vi "SpaceInvaders.vi"() -> ()   [LabVIEW 2022 SP3]
uses:
  TransPicture.ctl
  SelectKb.ctl
  ShipShootEnum.ctl
  InvaderPositionArray.ctl
  move_dir_lr.ctl
  ShotCluster.ctl
  move_dir_ud.ctl
  <vilib>/Utility/error.llb/Trim Whitespace One-Sided.vi
  Globals.vi
panel:
  out "ShootEnergy":dbl(slide) scale=0.0..500.0
  out "Intensity_DP":u8[][](graph)
  out "Ship":T1
  out "Invaders":T1
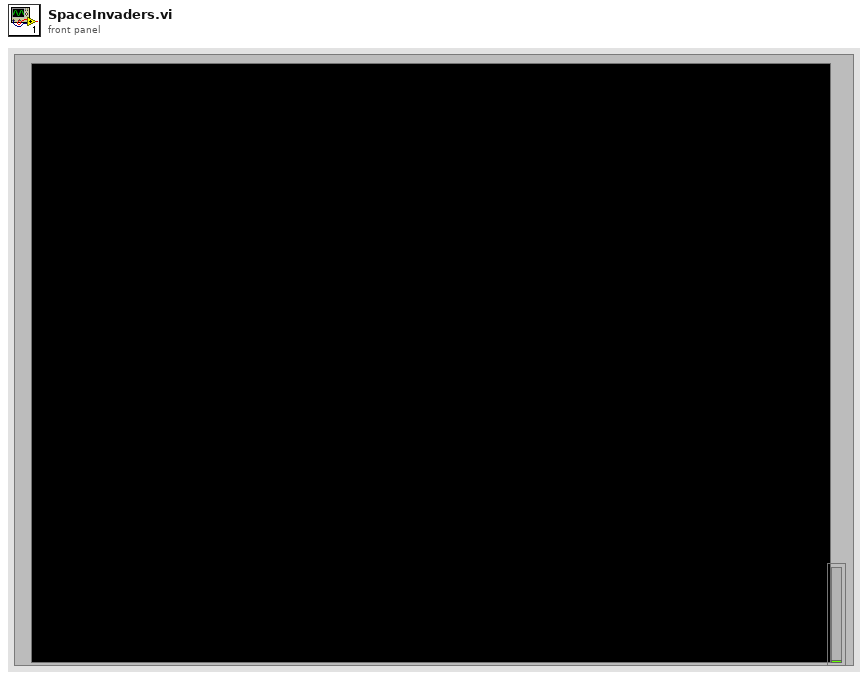
[diagram p1: front panel]
types:
  T1 = typedef "TransPicture.ctl" = picture
  T2 = typedef "ShipShootEnum.ctl" = enum16{"Init", "Read", "Reset"}
  T3 = typedef "SelectKb.ctl" = enum16{"InitKeyboard", "GetPressedKeys"}
  T4 = enum16{"0", "1", "2", "3", "4", "5", "6", "7", "8", "9", "A", "B", "C", "D", "E", "F", "G", "H", "I", "J", "K", "L", "M", "N", "O", "P", "Q", "R", "S", "T", "U", "V", "W", "X", "Y", "Z", "F1", "F2", "F3", "F4", "F5", "F6", "F7", "F8", "F9", "F10", "F11", "F12", "F13", "F14", "F15", "ADD", "BACK", "BACKSLASH", "CAPITAL", "COMMA", "DECIMAL", "DELETE", "DIVIDE", "DOWN", "END", "EQUALS", "ESCAPE", "GRAVE (`)", "HOME", "INSERT", "LBRACKET", "LCONTROL", "LEFT", "L ALT", "LSHIFT", "LWIN", "MINUS", "MULTIPLY", "NEXT", "NUMLOCK", "NUMPAD_0", "NUMPAD_1", "NUMPAD_2", "NUMPAD_3", "NUMPAD_4", "NUMPAD_5", "NUMPAD_6", "NUMPAD_7", "NUMPAD_8", "NUMPAD_9", "PAUSE", "PERIOD", "PRIOR (PG UP)", "RBRACKET", "RCONTROL", "RETURN", "RIGHT", "R ALT", "RSHIFT", "RWIN", "SCROLL", "SEMICOLON", "SLASH", "SPACE", "SUBTRACT", "TAB", "UP", "ENTER (num pad)", "' (quote)"}
  T5 = enum32{"Invalid", "Standard", "Closed", "Hidden", "Minimized", "Maximized"}
  T6 = enum32{"invalid app kind", "Development System", "Run Time System", "Student Edition", "Embedded LabVIEW", "Evaluation", "Custom"}
  T7 = typedef "move_dir_lr.ctl" = enum16{"right", "left"}
  T8 = typedef "InvaderPositionArray.ctl" = cluster{"InvaderAlive":bool[][], "InvaderPosArray":cluster{"left":i16, "top":i16, "right":i16, "bottom":i16}[][], "Direction":T7}
  T9 = typedef "move_dir_ud.ctl" = enum16{"up", "down"}
  T10 = typedef "ShotCluster.ctl" = cluster{"Speed":u32, "Length":u32, "Width":u32, "Position":cluster{"left":i16, "top":i16, "right":i16, "bottom":i16}, "Direction":T9}
  T11 = enum16{"0", "1", "2", "3", "4", "5", "6", "7", "8", "9", "A", "B", "C", "D", "E", "F", "G", "H", "I", "J", "K", "L", "M", "N", "O", "P", "Q", "R", "S", "T", "U", "V", "W", "X", "Y", "Z", "F1", "F2", "F3", "F4", "F5", "F6", "F7", "F8", "F9", "F10", "F11", "F12", "F13", "F14", "F15", "ADD", "BACK", "BACKSLASH", "CAPITAL", "COMMA", "DECIMAL", "DELETE", "DIVIDE", "DOWN", "END", "EQUALS", "ESCAPE", "GRAVE (`)", "HOME", "INSERT", "LBRACKET", "LCONTROL", "LEFT", "L ALT", "LSHIFT", "LWIN", "MINUS", "MULTIPLY", "NEXT", "NUMLOCK", "NUMPAD_0", "NUMPAD_1", "NUMPAD_2", "NUMPAD_3", "NUMPAD_4", "NUMPAD_5", "NUMPAD_6", "NUMPAD_7", "NUMPAD_8", "NUMPAD_9", "PAUSE", "PERIOD", "PRIOR (PG UP)", "RBRACKET", "RCONTROL", "RETURN", "RIGHT", "R ALT", "RSHIFT", "RWIN", "SCROLL", "SEMICOLON", "SLASH", "SPACE", "SUBTRACT", "TAB", "UP", "ENTER (num pad)", "' (quote)"}[]
  T12 = typedef "InitCluster.ctl" = cluster{"Invader":T13, "Spaceship":T13, "game_screen":refnum<vi>, "BasePicture":picture, "invader_screen":refnum<vi>, "InvaderPicPosition":T16, "Invader_down_speed":i16, "FPS":u16, "InvaderBlockSize":T17, "ship_screen":refnum<vi>, "ShipBlockSize":T17, "ShipPicPosition":T16, "LastUpdate":u32, "Intensity_Dp":refnum<vi>, "IntensityArray":u8[][], "ShotArray":T10[], "InvaderShotTimeArray":u32[], "ShootPeriod_ms":i32, "LastShipShot":u32}
  T13 = typedef "CharacterCluster.ctl" = cluster{"image":T14, "Width":u32, "Hieght":u32, "SpeedCharacter":u32, "Shot":T15, "IntensityArray":u8[][]}
  T14 = typedef "imagedata.ctl" = cluster{"image type":i32, "image depth":i32, "image":u8[], "mask":u8[], "colors":u32[], "Rectangle":cluster{"left":i16, "top":i16, "right":i16, "bottom":i16}}
  T15 = typedef "ShotInitCluster.ctl" = cluster{"Speed":u32, "Length":u32, "Width":u32}
  T16 = typedef "LVPositionTypeDef.ctl" = cluster{"Left":i32, "Top":i32}
  T17 = typedef "LVBoundsTypeDef.ctl" = cluster{"Width":u32, "Height":u32}
  T18 = cluster{"Core":cluster{"Current VI Reference":refnum<vi>, "Close Panel on Exit?":bool}, "InitCluster":T12, "InvaderPosArray":T8, "SpaceshipPosition":cluster{"left":i16, "top":i16, "right":i16, "bottom":i16}}
  T19 = cluster{"left":i16, "top":i16, "right":i16, "bottom":i16}
  T20 = cluster{"Current VI Reference":refnum<vi>, "Close Panel on Exit?":bool}
  T21 = cluster{"left":i16, "top":i16, "right":i16, "bottom":i16}[][]
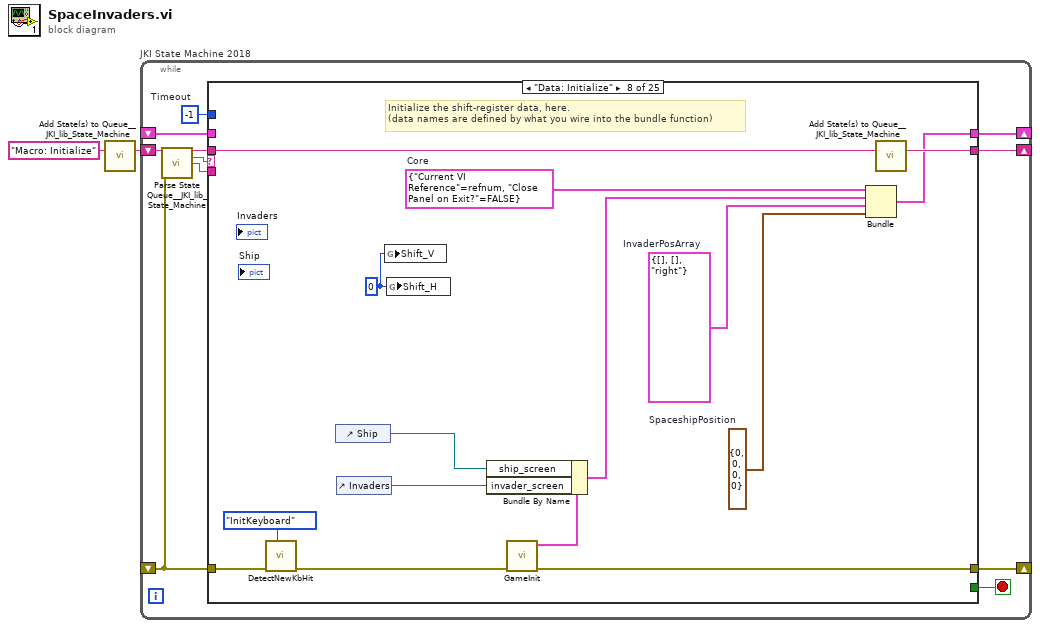
[diagram p0: block diagram]
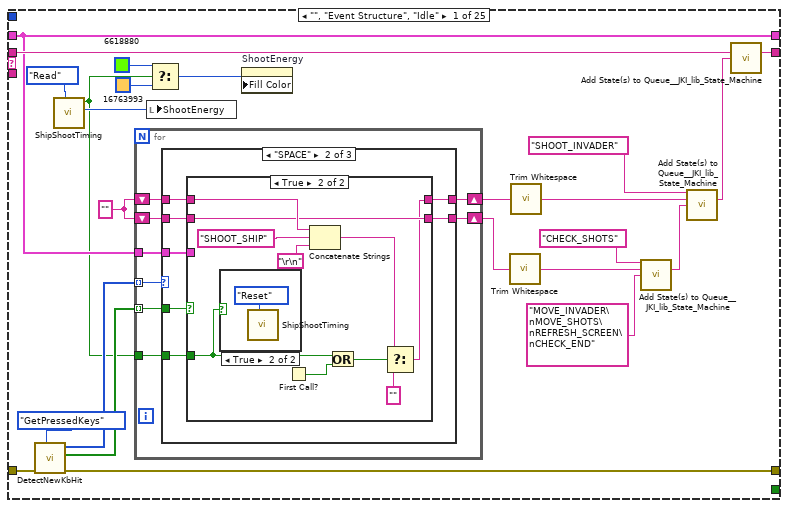
[diagram p2: hidden frame]
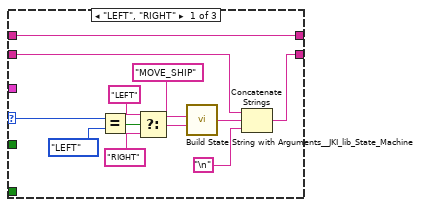
[diagram p3: hidden frame]
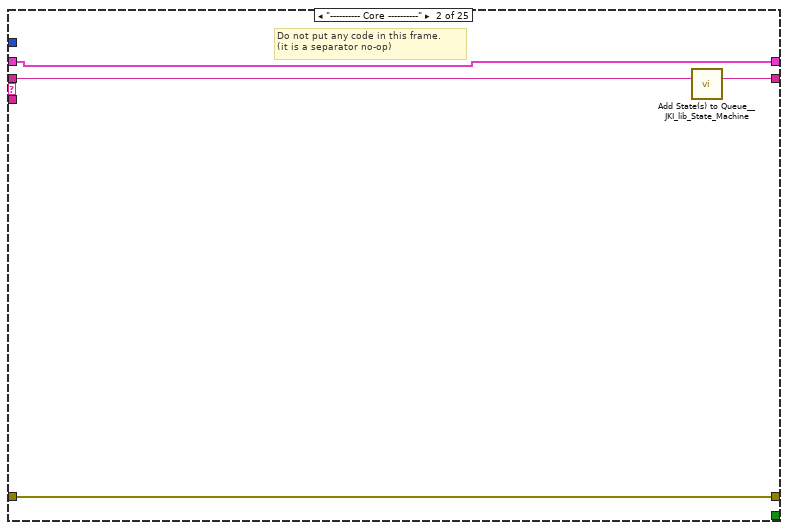
[diagram p7: hidden frame]
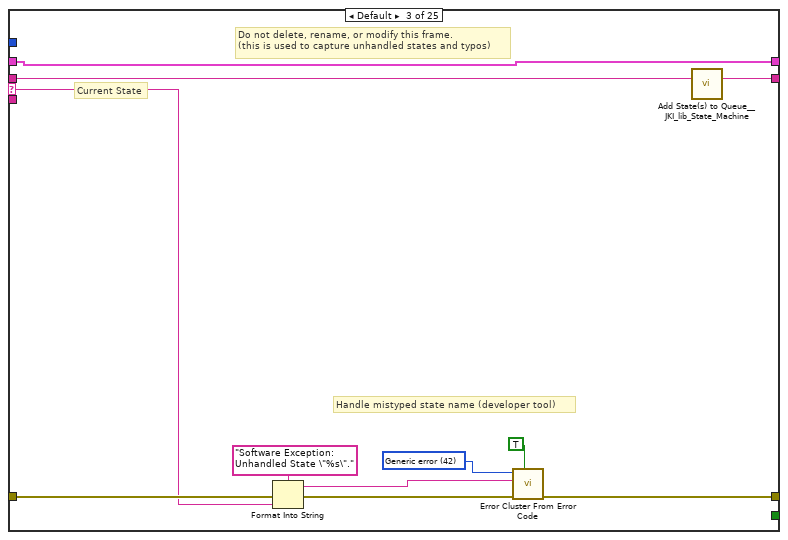
[diagram p8: hidden frame]
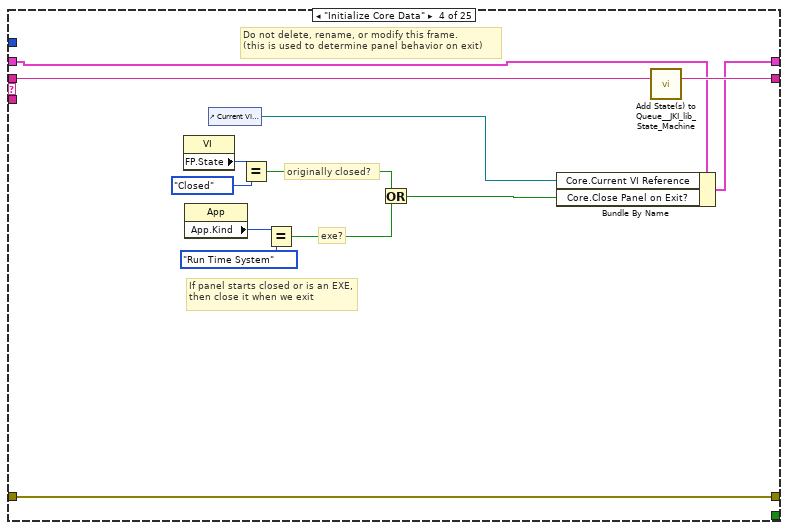
[diagram p9: hidden frame]
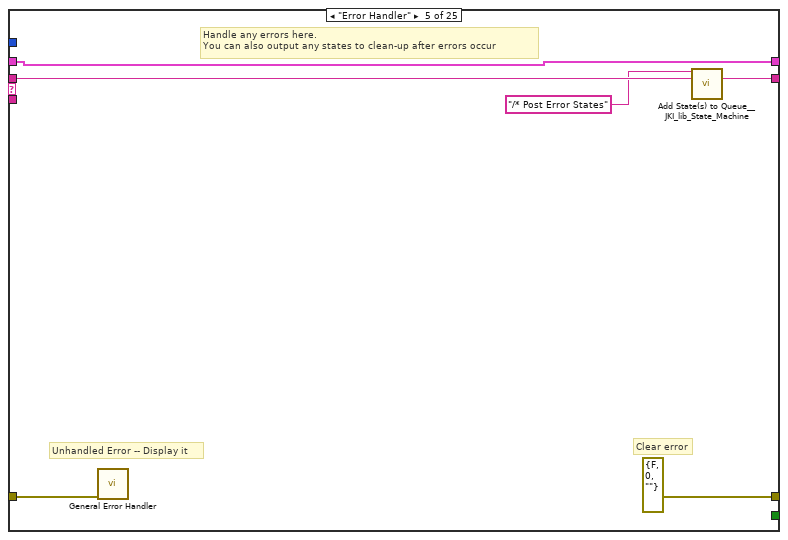
[diagram p10: hidden frame]
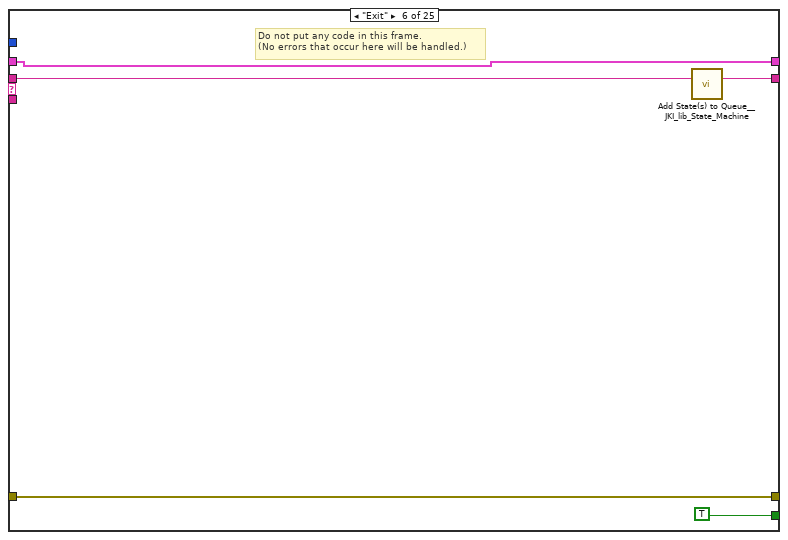
[diagram p11: hidden frame]
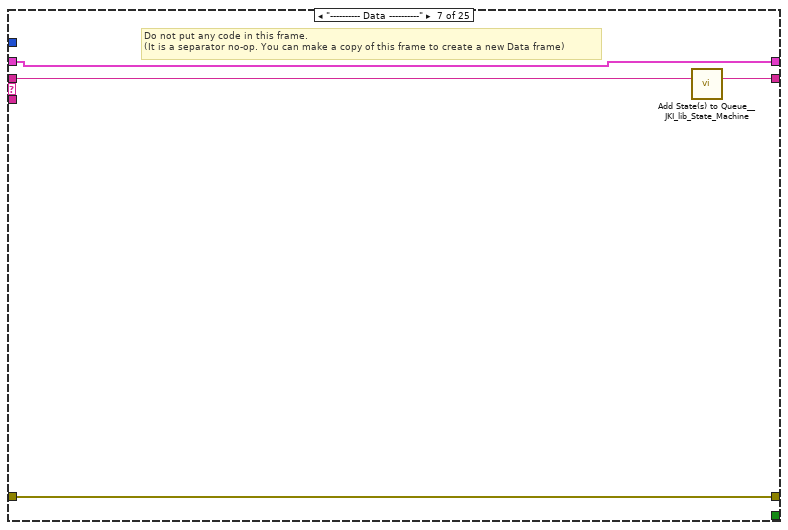
[diagram p12: hidden frame]
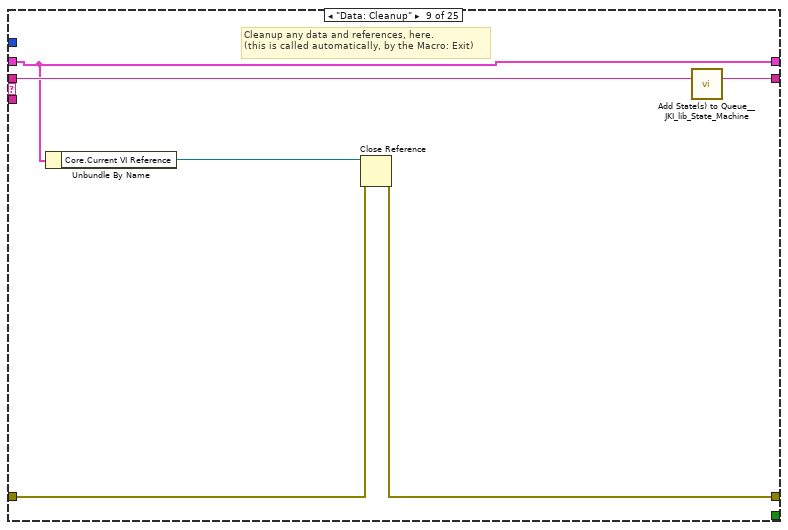
[diagram p13: hidden frame]
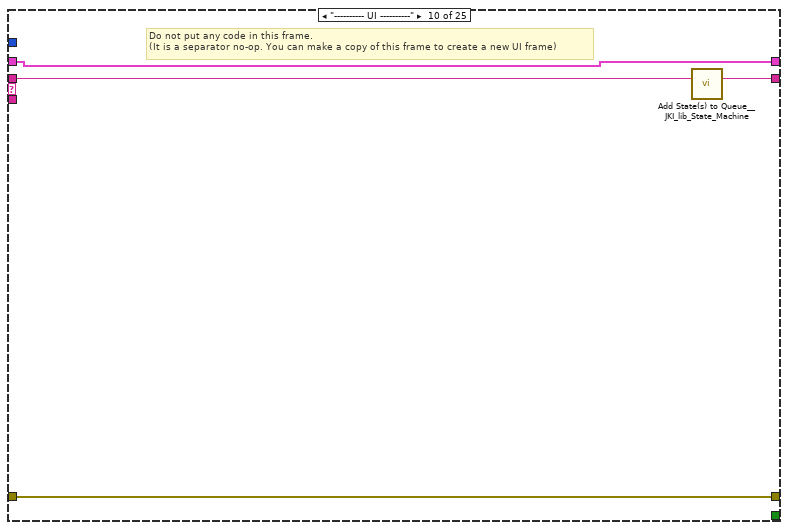
[diagram p14: hidden frame]
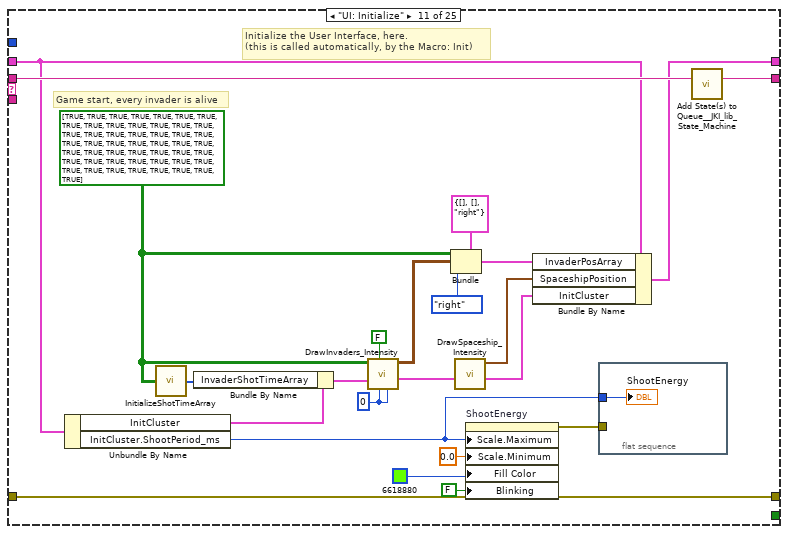
[diagram p15: hidden frame]
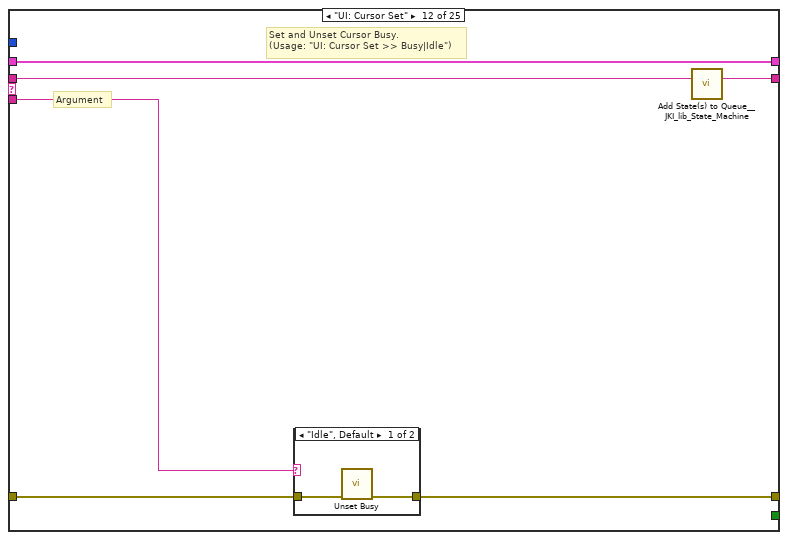
[diagram p16: hidden frame]
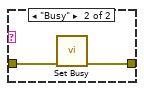
[diagram p17: hidden frame]
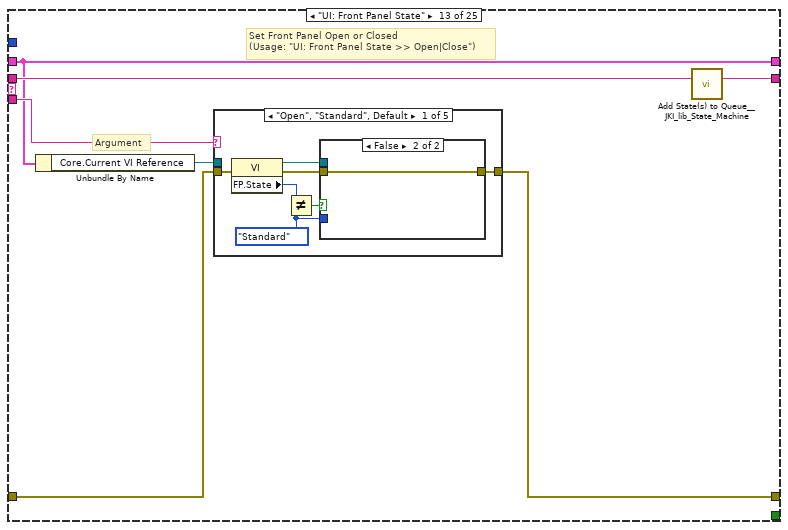
[diagram p18: hidden frame]
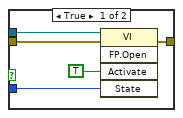
[diagram p19: hidden frame]
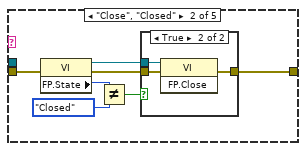
[diagram p20: hidden frame]
diagram:
  n1 = call <vilib>:"Add State(s) to Queue__JKI_lib_State_Machine.vi"("State(s) in (\"\")"="Macro: Initialize") -> ("States Out"=w2:string)  [unwired: 14 in]
  n2 = while "JKI State Machine 2018" {
    shift-right: [w6] -> _
    shift-left: _ -> [w3]
    shift-right: [w9] -> _
    shift-left: _ -> [w4]
    shift-right: [w8] -> _
    shift-left: w2 -> [w10]
    stop <- w7 stop-if-true
    w5 = -1  # Timeout
    n3 = call <vilib>:"Parse State Queue__JKI_lib_State_Machine.vi"("State Queue"=w10, "Error In (no error)"=w4) -> ("Remaining States"=w12:string, "Current State"=w13:string, "Arguments"=w11:string)  [unwired: 11 in]
    n4 = case shown="\"Data: Initialize\"" w13 {
      selector: w13 -> [_ _ w85 _ _ _ _ _ _ _ _ _ _ _ _ _ _ _ _ _ _ _ _ _ _]
      tunnel: w12 -> [w36 w83 w88 w107 w113 w118 w122 w137 w143 w147 w170 w177 w188 w252 w257 w267 w271 w282 w301 w306 w312 w321 w346 w366 w372]
      tunnel: w11 -> [_ _ _ _ _ _ _ _ _ _ _ w173 w183 _ _ _ _ _ _ _ w307 _ _ _ w373]
      tunnel: [w37 w81 w90 w105 errorcluster {"status"=FALSE, "code"=0, "source"=""} ("error out") w116 w120 w130 w140 w145 w159 w174 w185 w250 w255 w265 w269 w280 w299 w304 w310 w319 w344 w364 w377] -> w9
      tunnel: w4 -> [w32 w81 w89 w105 w110 w116 w120 w128 w141 w145 w159 w175 w186 w250 w255 w265 w269 w280 w299 w304 w310 w319 w344 w364 w377]
      tunnel: [w31 w82 w87 w106 w112 w117 w121 w136 w142 w146 w169 w176 w187 w251 w256 w266 w270 w281 w300 w305 w311 w320 w345 w365 w378] -> w8
      tunnel: [_ _ _ _ _ TRUE _ _ _ _ _ _ _ _ _ _ _ _ _ _ _ _ _ _ _] -> w7
      tunnel: [w20 w80 w84 w95 w108 w114 w119 w126 w139 w144 w165 w172 w182 w249 w253 w259 w268 w278 w298 w302 w308 w313 w332 w363 w376] -> w6
      tunnel: w5 -> [_ _ _ _ _ _ _ _ _ _ _ _ _ _ _ _ _ _ _ _ _ _ _ _ _]
      tunnel: w3 -> [w20 w80 w84 w96 w108 w114 w119 _ w139 w144 w162 w172 w182 w249 w253 w259 w268 w279 w297 w303 w309 w316 w343 w349 w376]
      frame "", "Event Structure", "Idle" {
        w27 = ""
        n5 = call "DetectNewKbHit.vi"("SelectKb"=SelectKb."GetPressedKeys", "error in"=w32) -> ("error out"=w37:errorcluster, "NewKey"=w34:bool[], "keys pressed"=w33:T11)  [unwired: 7 in]
        n6 = call "ShipShootTiming.vi"("Selector"=ShipShootEnum."Read") -> ("Time"=w18:u32, "Ready2Shoot"=w17:bool)  [unwired: 9 in]
        n7 = for {
          tunnel: w33 -> [w45] mode=indexing
          tunnel: w34 -> [w44] mode=indexing
          shift-right: [w42] -> w35
          shift-left: w27 -> [w43]
          shift-right: [w40] -> w26
          shift-left: w27 -> [w41]
          tunnel: w20 -> [w39]
          tunnel: w17 -> [w38]
          n8 = case shown="\"SPACE\"" w45 {
            selector: w45 -> [w57 _ _]
            tunnel: w44 -> [_ w64 _]
            tunnel: w43 -> [w48 w63 w79]
            tunnel: [w49 w62 w79] -> w42
            tunnel: w41 -> [w46 w61 w78]
            tunnel: [w46 w60 w78] -> w40
            tunnel: w39 -> [_ w59 _]
            tunnel: w38 -> [_ w58 _]
            frame "LEFT", "RIGHT" {
              n9 = Equal?(x=w57, y=T4."LEFT" ("keyType 3")) -> (x = y?=w55:bool)
              n10 = Select(t="LEFT", s=w55, f="RIGHT") -> (s? t:f=w53:string)
              n11 = call <vilib>:"Build State String with Arguments__JKI_lib_State_Machine.vi"("Arguments (\"\")"=w53, "State"="MOVE_SHIP") -> ("State with Arguments"=w47:string)  [unwired: 4 in]
              n12 = Concatenate Strings(w48, w47, "\n") -> (w49:string)
            }
            frame "SPACE" {
              n13 = case shown="True" w64 {
                tunnel: w63 -> [w66 w73]
                tunnel: [w66 w73] -> w62
                tunnel: w61 -> [w65 w74]
                tunnel: [w65 w70] -> w60
                tunnel: w59 -> [_ _]
                tunnel: w58 -> [_ w67]
                frame False {
                }
                frame True {
                  n14 = case shown="True" w67 {
                    frame False {
                    }
                    frame True {
                      n15 = call "ShipShootTiming.vi"("Selector"=ShipShootEnum."Reset") -> ()  [unwired: 9 in, 2 out]
                    }
                  }
                  n16 = First Call?() -> (First Call?: T/F=w69:bool)
                  n17 = Concatenate Strings(w74, "SHOOT_SHIP" ("string"), "\r\n") -> (w72:string)
                  n18 = Or(x=w67, y=w69) -> (x .or. y?=w68:bool)
                  n19 = Select(t=w72, s=w68, f="") -> (s? t:f=w70:string)
                }
              }
            }
            frame Default {
            }
          }
        }
        n20 = local write "ShootEnergy"(w18) -> ()
        n21 = Select(t=u32 6618880, s=w17, f=u32 16763993) -> (s? t:f=w14:u32)
        n22 = property on="ShootEnergy" class="Slide (strict)"("Fill Color"=w14) -> ()  [unwired: 2 in, 2 out]
        n23 = call <vilib>:"Trim Whitespace.vi"("string"=w35) -> ("trimmed string"=w23:string)  [unwired: 1 in]
        n24 = call <vilib>:"Trim Whitespace.vi"("string"=w26) -> ("trimmed string"=w25:string)  [unwired: 1 in]
        n25 = call <vilib>:"Add State(s) to Queue__JKI_lib_State_Machine.vi"("State(s) in Front (\"\")"="CHECK_SHOTS" ("State(s) at Back (\"\")"), "State(s) in (\"\")"=w23, "State(s) at Back (\"\")"="MOVE_INVADER\nMOVE_SHOTS\nREFRESH_SCREEN\nCHECK_END" ("State(s) at Back (\"\")")) -> ("States Out"=w22:string)  [unwired: 12 in]
        n26 = call <vilib>:"Add State(s) to Queue__JKI_lib_State_Machine.vi"("State(s) in Front (\"\")"="SHOOT_INVADER", "State(s) in (\"\")"=w25, "State(s) at Back (\"\")"=w22) -> ("States Out"=w30:string)  [unwired: 12 in]
        n27 = call <vilib>:"Add State(s) to Queue__JKI_lib_State_Machine.vi"("State(s) in (\"\")"=w36, "State(s) at Back (\"\")"=w30) -> ("States Out"=w31:string)  [unwired: 13 in]
      }
      frame "---------- Core ----------" {
        # "Do not put any code in this frame.\n(it is a separator no-op)"
        n28 = call <vilib>:"Add State(s) to Queue__JKI_lib_State_Machine.vi"("State(s) in (\"\")"=w83) -> ("States Out"=w82:string)  [unwired: 14 in]
      }
      frame Default {
        w93 = 42 items=["No error", "Argument error", "Memory is full", "Out of zone", "End of file", "File already open", "Generic file I/O error", "File not found", "File permission error", "Disk is full", "Duplicate path", "Too many files open", "System feature not enabled", "Resource file not found", "Cannot add resource", "Resource not found", "Image not found", "Image memory error", "Pen does not exist", "Config type invalid", "Config token not found", "Config parse error", "Config memory error", "Bad external code format", "Bad external code offset", "External code not present", "Null window", "Destroy window error", "Null menu", "Print aborted", "Bad print record", "Print driver error", "Windows error during printing", "Memory error during printing", "Print dialog error", "Generic print error", "Invalid device refnum", "Device not found", "Device parameter error", "Device unit error", "Cannot open device", "Device call aborted", "Generic error", "Cancelled by user", "Object ID too low", "Object ID too high", "Object not in heap", "Unknown heap", "Unknown object (invalid DefProc)", "Unknown object (DefProc not in table)", "Message out of range", "Invalid (null) method", "Unknown message", "Manager call not supported", "Bad address", "Network operation in progress", "Network operation timed out", "Connection is busy", "Network attribute not supported", "Network error", "Address in use", "System out of memory", "Connection aborted", "Connection refused", "Not connected", "Already connected", "Connection closed", "Initialization error (interapplication manager)", "Bad occurrence", "Wait on unbound occurrence handler", "Occurrence queue overflow", "Datalog type conflict", "Unused", "Unrecognized type (interapplication manager)", "Memory corrupt", "Failed to make temporary DLL", "Old CIN version", "Drag socket not found", "Failed to load drop-object", "Failed to register OLE object", "Failed to release OLE object", "Format specifier type mismatch", "Unknown format specifier", "Too few format specifiers", "Too many format specifiers", "Scan failed", "Newer CIN version", "Error converting to variant", "Runtime menu error", "Password tampered", "Variant attribute not found", "Incompatible variant data type", "Event data is not available", "Event Store is not present", "Occurrence is not found", "Event Queue is not created", "Event info is not available", "Refnum passed is NULL", "Error retrieving Class GUID", "Error retrieving CoClass GUID", "Error retrieving TypeLib GUID.", "Bad built application magic bytes.", "Specific driver is different from the specific driver associated with the Logical Name.", "There is no session opened to the class driver.", "Max Error", "MAX - Error with config objects", "MAX - Error loading configuration", "MAX - Group not supported"]
        # "Current State"
        # "Do not delete, rename, or modify this frame.\n(this is used to capture unhandled states and typos)"
        # "Handle mistyped state name (developer tool)"
        n29 = Format Into String(format string="Software Exception: Unhandled State \"%s\"." ("message"), error in=w89, w85) -> (resulting string=w92:string, error out=w91:errorcluster)  [unwired: 1 in]
        n30 = call <vilib>:"Error Cluster From Error Code.vi"("show call chain? (False)"=TRUE, "error in (no error)"=w91, "error message (\"\")"=w92, "error code (0)"=w93) -> ("error out"=w90:errorcluster)  [unwired: 5 in]
        n31 = call <vilib>:"Add State(s) to Queue__JKI_lib_State_Machine.vi"("State(s) in (\"\")"=w88) -> ("States Out"=w87:string)  [unwired: 14 in]
      }
      frame "Initialize Core Data" {
        # "Do not delete, rename, or modify this frame.\n(this is used to determine panel behavior on exit)"
        # "originally closed?"
        # "exe?"
        # "If panel starts closed or is an EXE, then close it when we exit"
        n32 = property class="VI"() -> ("FP.State"=w99:T5)  [unwired: 2 in, 2 out]
        n33 = property class="App"() -> ("App.Kind"=w104:T6)  [unwired: 2 in, 2 out]
        n34 = control-ref of="Current VI Reference"() -> (w100:refnum<vi>)
        n35 = Equal?(x=w99, y=T5."Closed" ("Front Panel Window:State")) -> (x = y?=w97:bool)
        n36 = Equal?(x=w104, y=T6."Run Time System" ("Application:Kind")) -> (x = y?=w102:bool)
        n37 = Or(x=w97, y=w102) -> (x .or. y?=w101:bool)
        n38 = Bundle By Name(cluster=w96, "Core.Current VI Reference"=w100, "Core.Close Panel on Exit?"=w101) -> (w95:T18)
        n39 = call <vilib>:"Add State(s) to Queue__JKI_lib_State_Machine.vi"("State(s) in (\"\")"=w107) -> ("States Out"=w106:string)  [unwired: 14 in]
      }
      frame "Error Handler" {
        # "Unhandled Error -- Display it"
        # "Handle any errors here.\nYou can also output any states to clean-up after errors occur"
        # "Clear error"
        n40 = call <vilib>:"General Error Handler.vi"("error in (no error)"=w110) -> ()  [unwired: 10 in, 5 out]
        n41 = call <vilib>:"Add State(s) to Queue__JKI_lib_State_Machine.vi"("State(s) in Front (\"\")"="/* Post Error States", "State(s) in (\"\")"=w113) -> ("States Out"=w112:string)  [unwired: 13 in]
      }
      frame "Exit" {
        # "Do not put any code in this frame.\n(No errors that occur here will be handled.)"
        n42 = call <vilib>:"Add State(s) to Queue__JKI_lib_State_Machine.vi"("State(s) in (\"\")"=w118) -> ("States Out"=w117:string)  [unwired: 14 in]
      }
      frame "---------- Data ----------" {
        # "Do not put any code in this frame.\n(It is a separator no-op. You can make a copy of this frame to create a new Data frame)"
        n43 = call <vilib>:"Add State(s) to Queue__JKI_lib_State_Machine.vi"("State(s) in (\"\")"=w122) -> ("States Out"=w121:string)  [unwired: 14 in]
      }
      frame "Data: Initialize" {
        w123 = i16 0 ("Shift_H")
        w131 = T19 {"left"=0, "top"=0, "right"=0, "bottom"=0}  # SpaceshipPosition
        w132 = T8 {"InvaderAlive"=[], "InvaderPosArray"=[], "Direction"=enum."right"}  # InvaderPosArray
        w135 = T20 {"Current VI Reference"=refnum, "Close Panel on Exit?"=FALSE}  # Core
        # "Initialize the shift-register data, here.\n(data names are defined by what you wire into the bundle function)"
        n44 = call "DetectNewKbHit.vi"("SelectKb"=SelectKb."InitKeyboard", "error in"=w128) -> ("error out"=w129:errorcluster)  [unwired: 7 in, 2 out]
        n45 = control-ref of="Ship"() -> (w124:refnum<vi>)
        n46 = control-ref of="Invaders"() -> (w125:refnum<vi>)
        n47 = global write "Globals.vi" "Shift_V"(w123) -> ()
        n48 = global write "Globals.vi" "Shift_H"(w123) -> ()
        n49 = call "GameInit.vi"("error in"=w129) -> ("error out"=w130:errorcluster, "InitCluster"=w134:T12)  [unwired: 9 in]
        n50 = Bundle By Name(cluster=w134, "ship_screen"=w124, "invader_screen"=w125) -> (w133:T12)
        n51 = Bundle("Core"=w135, "InitCluster"=w133, "InvaderPosArray"=w132, "SpaceshipPosition"=w131) -> (w126:T18)  [unwired: 1 in]
        n52 = call <vilib>:"Add State(s) to Queue__JKI_lib_State_Machine.vi"("State(s) in (\"\")"=w137) -> ("States Out"=w136:string)  [unwired: 14 in]
      }
      frame "Data: Cleanup" {
        # "Cleanup any data and references, here.\n(this is called automatically, by the Macro: Exit)"
        n53 = Unbundle By Name(w139) -> ("Core.Current VI Reference"=w138:refnum<vi>)
        n54 = Close Reference(reference=w138, error in (no error)=w141) -> (error out=w140:errorcluster)
        n55 = call <vilib>:"Add State(s) to Queue__JKI_lib_State_Machine.vi"("State(s) in (\"\")"=w143) -> ("States Out"=w142:string)  [unwired: 14 in]
      }
      frame "---------- UI ----------" {
        # "Do not put any code in this frame.\n(It is a separator no-op. You can make a copy of this frame to create a new UI frame)"
        n56 = call <vilib>:"Add State(s) to Queue__JKI_lib_State_Machine.vi"("State(s) in (\"\")"=w147) -> ("States Out"=w146:string)  [unwired: 14 in]
      }
      frame "UI: Initialize" {
        w163 = 0 ("Step_V")
        w154 = bool[][] [[TRUE, TRUE, TRUE, TRUE, TRUE, TRUE, TRUE, TRUE, TRUE, TRUE], [TRUE, TRUE, TRUE, TRUE, TRUE, TRUE, TRUE, TRUE, TRUE, TRUE], [TRUE, TRUE, TRUE, TRUE, TRUE, TRUE, TRUE, TRUE, TRUE, TRUE], [TRUE, TRUE, TRUE, TRUE, TRUE, TRUE, TRUE, TRUE, TRUE, TRUE], [TRUE, TRUE, TRUE, TRUE, TRUE, TRUE, TRUE, TRUE, TRUE, TRUE]]
        # "Game start, every invader is alive"
        # "Initialize the User Interface, here.\n(this is called automatically, by the Macro: Init)"
        n57 = Unbundle By Name(w162) -> ("InitCluster"=w156:T12, "InitCluster.ShootPeriod_ms"=w151:i32)
        n58 = call "InitializeShotTimeArray.vi"("InvaderArray"=w154) -> ("InvaderColoumnTimeArray"=w155:u32[])
        n59 = Bundle By Name(cluster=w156, "InvaderShotTimeArray"=w155) -> (w157:T12)
        n60 = call "DrawInvaders_Intensity.vi"("Step_V"=w163, "Step_H"=w163, "Clear"=FALSE, "InitCluster_IN"=w157, "InvaderArray"=w154) -> ("InitCluster_OUT"=w161:T12, "InvaderPosArray"=w168:T21)  [unwired: 5 in]
        n61 = Bundle(cluster=T8 {"InvaderAlive"=[], "InvaderPosArray"=[], "Direction"=enum."right"} ("InvaderPosArray"), "InvaderAlive"=w154, "InvaderPosArray"=w168, "Direction"=move_dir_lr."right") -> (w166:T8)
        n62 = call "DrawSpaceship_Intensity.vi"("InitCluster_IN"=w161) -> ("InitCluster_OUT"=w158:T12, "spaceship_position"=w160:T19)  [unwired: 9 in]
        n63 = property on="ShootEnergy" class="Slide (strict)"("Scale.Maximum"=w151, "Scale.Minimum"=0.0 ("Scale.Range:Minimum"), "Fill Color"=u32 6618880, "Blinking"=FALSE) -> (error out=w152:errorcluster)  [unwired: 2 in, 1 out]
        n64 = Bundle By Name(cluster=w162, "InvaderPosArray"=w166, "SpaceshipPosition"=w160, "InitCluster"=w158) -> (w165:T18)
        n65 = flat-sequence {
          tunnel: w152 -> [_]
          tunnel: w151 -> [w171]
          frame #0 {
            "ShootEnergy" <- w171
          }
        }
        n66 = call <vilib>:"Add State(s) to Queue__JKI_lib_State_Machine.vi"("State(s) in (\"\")"=w170) -> ("States Out"=w169:string)  [unwired: 14 in]
      }
      frame "UI: Cursor Set" {
        # "Argument"
        # "Set and Unset Cursor Busy.\n(Usage: \"UI: Cursor Set >> Busy|Idle\")"
        n67 = case shown="\"Idle\", Default" w173 {
          tunnel: w175 -> [w179 w181]
          tunnel: [w178 w180] -> w174
          frame "Idle", Default {
            n68 = call <vilib>:"Unset Busy.vi"("error in (no error)"=w179) -> ("error out"=w178:errorcluster)  [unwired: 10 in]
          }
          frame "Busy" {
            n69 = call <vilib>:"Set Busy.vi"("error in (no error)"=w181) -> ("error out"=w180:errorcluster)  [unwired: 9 in, 1 out]
          }
        }
        n70 = call <vilib>:"Add State(s) to Queue__JKI_lib_State_Machine.vi"("State(s) in (\"\")"=w177) -> ("States Out"=w176:string)  [unwired: 14 in]
      }
      frame "UI: Front Panel State" {
        # "Argument"
        # "Set Front Panel Open or Closed\n(Usage: \"UI: Front Panel State >> Open|Close\")"
        n71 = Unbundle By Name(w182) -> ("Core.Current VI Reference"=w184:refnum<vi>)
        n72 = case shown="\"Open\", \"Standard\", Default" w183 {
          tunnel: w186 -> [w194 w207 w218 w230 w242]
          tunnel: [w195 w208 w219 w231 w243] -> w185
          tunnel: w184 -> [_ _ _ _ _]
          frame "Open", "Standard", Default {
            w189 = T5."Standard" ("State")
            n73 = property class="VI"(error in=w194) -> (reference out=w192:refnum<vi>, error out=w193:errorcluster, "FP.State"=w191:T5)  [unwired: 1 in]
            n74 = Not Equal?(x=w191, y=w189) -> (x != y?=w190:bool)
            n75 = case shown="False" w190 {
              tunnel: [w199 w201] -> w195
              tunnel: w193 -> [w198 w201]
              tunnel: w192 -> [w197 _]
              tunnel: w189 -> [w196 _]
              frame True {
                n76 = invoke class="VI" method="FP.Open"(reference=w197, error in=w198, "Activate"=TRUE, "State"=w196) -> (error out=w199:errorcluster)  [unwired: 1 in, 4 out]
              }
              frame False {
              }
            }
          }
          frame "Close", "Closed" {
            n77 = property class="VI"(error in=w207) -> (reference out=w205:refnum<vi>, error out=w206:errorcluster, "FP.State"=w203:T5)  [unwired: 1 in]
            n78 = Not Equal?(x=w203, y=T5."Closed" ("Front Panel Window:State")) -> (x != y?=w202:bool)
            n79 = case shown="True" w202 {
              tunnel: [w209 w212] -> w208
              tunnel: w206 -> [w209 w211]
              tunnel: w205 -> [_ w210]
              frame False {
              }
              frame True {
                n80 = invoke class="VI" method="FP.Close"(reference=w210, error in=w211) -> (error out=w212:errorcluster)  [unwired: 1 in, 2 out]
              }
            }
          }
          frame "Hidden", "Hide" {
            w213 = T5."Hidden" ("State")
            n81 = property class="VI"(error in=w218) -> (reference out=w216:refnum<vi>, error out=w217:errorcluster, "FP.State"=w215:T5)  [unwired: 1 in]
            n82 = Not Equal?(x=w215, y=w213) -> (x != y?=w214:bool)
            n83 = case shown="True" w214 {
              tunnel: [w223 w224] -> w219
              tunnel: w217 -> [w222 w224]
              tunnel: w216 -> [w221 _]
              tunnel: w213 -> [w220 _]
              frame True {
                n84 = invoke class="VI" method="FP.Open"(reference=w221, error in=w222, "State"=w220) -> (error out=w223:errorcluster)  [unwired: 2 in, 4 out]
              }
              frame False {
              }
            }
          }
          frame "Minimize", "Minimized" {
            w225 = T5."Minimized" ("State")
            n85 = property class="VI"(error in=w230) -> (reference out=w228:refnum<vi>, error out=w229:errorcluster, "FP.State"=w227:T5)  [unwired: 1 in]
            n86 = Not Equal?(x=w227, y=w225) -> (x != y?=w226:bool)
            n87 = case shown="True" w226 {
              tunnel: [w235 w236] -> w231
              tunnel: w229 -> [w234 w236]
              tunnel: w228 -> [w233 _]
              tunnel: w225 -> [w232 _]
              frame True {
                n88 = invoke class="VI" method="FP.Open"(reference=w233, error in=w234, "State"=w232) -> (error out=w235:errorcluster)  [unwired: 2 in, 4 out]
              }
              frame False {
              }
            }
          }
          frame "Maximize", "Maximized" {
            w237 = T5."Maximized" ("State")
            n89 = property class="VI"(error in=w242) -> (reference out=w240:refnum<vi>, error out=w241:errorcluster, "FP.State"=w239:T5)  [unwired: 1 in]
            n90 = Not Equal?(x=w239, y=w237) -> (x != y?=w238:bool)
            n91 = case shown="True" w238 {
              tunnel: [w247 w248] -> w243
              tunnel: w241 -> [w246 w248]
              tunnel: w240 -> [w245 _]
              tunnel: w237 -> [w244 _]
              frame True {
                n92 = invoke class="VI" method="FP.Open"(reference=w245, error in=w246, "State"=w244) -> (error out=w247:errorcluster)  [unwired: 2 in, 4 out]
              }
              frame False {
              }
            }
          }
        }
        n93 = call <vilib>:"Add State(s) to Queue__JKI_lib_State_Machine.vi"("State(s) in (\"\")"=w188) -> ("States Out"=w187:string)  [unwired: 14 in]
      }
      frame "---------- Macro ----------" {
        # "Do not put any code in this frame.\n(It is a separator no-op. You can make a copy of this frame to create a new Macro frame)"
        n94 = call <vilib>:"Add State(s) to Queue__JKI_lib_State_Machine.vi"("State(s) in (\"\")"=w252) -> ("States Out"=w251:string)  [unwired: 14 in]
      }
      frame "Macro: Initialize" {
        w254 = "Data: Initialize\nInitialize Core Data\nUI: Initialize\nUI: Front Panel State >> Open"  # Data: Initialize Initialize Core Data UI: Initialize UI: Front Panel State >> Open
        # "Initialization Macro\n(This is called once, when the VI starts)"
        n95 = call <vilib>:"Add State(s) to Queue__JKI_lib_State_Machine.vi"("State(s) in Front (\"\")"=w254, "State(s) in (\"\")"=w257) -> ("States Out"=w256:string)  [unwired: 13 in]
      }
      frame "Macro: Exit" {
        # "Exit Macro\n(This is called once, when the VI exits)"
        n96 = Unbundle By Name(w259) -> ("Core.Close Panel on Exit?"=w258:bool)
        n97 = Select(t="UI: Front Panel State >> Close", s=w258, f="") -> (s? t:f=w262:string)
        n98 = call <vilib>:"Add State(s) to Queue__JKI_lib_State_Machine.vi"("State(s) in (\"\")"=w262, "State(s) at Back (\"\")"="Data: Cleanup\nExit") -> ("States Out"=w260:string)  [unwired: 13 in]
        n99 = call <vilib>:"Add State(s) to Queue__JKI_lib_State_Machine.vi"("State(s) in Front (\"\")"=w260, "State(s) in (\"\")"=w267) -> ("States Out"=w266:string)  [unwired: 13 in]
      }
      frame "---------- New Category ----------" {
        # "Template Separator\n(You can make a copy of, or modify, this frame)"
        n100 = call <vilib>:"Add State(s) to Queue__JKI_lib_State_Machine.vi"("State(s) in (\"\")"=w271) -> ("States Out"=w270:string)  [unwired: 14 in]
      }
      frame "REFRESH_SCREEN" {
        # "Template Separator\n(You can make a copy of, or modify, this frame)"
        n101 = Unbundle By Name(w279) -> ("InitCluster.IntensityArray"=w272:u8[][], "InitCluster.FPS"=w275:u16, "InitCluster.LastUpdate"=w277:u32)  [unwired: 1 out]
        n102 = flat-sequence {
          tunnel: w277 -> [w288]
          tunnel: w275 -> [w283]
          tunnel: [w284] -> w274
          tunnel: w274 -> [w293]
          tunnel: [w294] -> w276
          tunnel: w272 -> [w296]
          tunnel: [w295] -> w273
          tunnel: w276 -> [w295]
          frame #0 {
            n103 = Tick Count (ms)() -> (millisecond timer value=w291:u32)
            n104 = Divide(x=u32 1000, y=w283) -> (x/y=w290:dbl)
            n105 = Subtract(x=w291, y=w288) -> (x-y=w289:u32)
            n106 = First Call?() -> (First Call?: T/F=w287:bool)
            n107 = Subtract(x=w290, y=w289) -> (x-y=w286:dbl)
            n108 = Select(t=0.0, s=w287, f=w286) -> (s? t:f=w284:dbl)
          }
          frame #1 {
            n109 = Wait (ms)(milliseconds to wait=w293) -> ()  [unwired: 1 out]
          }
          frame #2 {
            n110 = Tick Count (ms)() -> (millisecond timer value=w294:u32)
          }
          frame #3 {
            "Intensity_DP" <- w296
          }
        }
        n111 = Bundle By Name(cluster=w279, "InitCluster.LastUpdate"=w273) -> (w278:T18)
        n112 = call <vilib>:"Add State(s) to Queue__JKI_lib_State_Machine.vi"("State(s) in (\"\")"=w282) -> ("States Out"=w281:string)  [unwired: 14 in]
      }
      frame "MOVE_INVADER" {
        n113 = call "move_invader.vi"("MainCluster_IN"=w297) -> ("MainCluster_OUT"=w298:T18)
        n114 = call <vilib>:"Add State(s) to Queue__JKI_lib_State_Machine.vi"("State(s) in (\"\")"=w301) -> ("States Out"=w300:string)  [unwired: 14 in]
      }
      frame "SHOOT_INVADER" {
        n115 = call "FindShootingInvaders.vi"("MainCluster_IN"=w303) -> ("MainCluster_OUT"=w302:T18)
        n116 = call <vilib>:"Add State(s) to Queue__JKI_lib_State_Machine.vi"("State(s) in (\"\")"=w306) -> ("States Out"=w305:string)  [unwired: 14 in]
      }
      frame "MOVE_SHIP" {
        n117 = call "MoveShip.vi"("MainCluster_IN"=w309, "Direction"=w307) -> ("MainCluster _OUT"=w308:T18)
        n118 = call <vilib>:"Add State(s) to Queue__JKI_lib_State_Machine.vi"("State(s) in (\"\")"=w312) -> ("States Out"=w311:string)  [unwired: 14 in]
      }
      frame "MOVE_SHOTS" {
        n119 = Unbundle By Name(w316) -> ("InitCluster.ShotArray"=w318:T10[], "InitCluster.IntensityArray"=w317:u8[][])
        n120 = for {
          tunnel: w318 -> [w326] mode=indexing
          shift-right: [w324] -> w314
          shift-left: w317 -> [w325]
          tunnel: [w323] -> w315 mode=indexing
          n121 = call "DrawShots.vi"("Clear"=TRUE, "IntensityArray_IN"=w325, "Shot"=w326) -> ("IntensityArray_OUT"=w324:u8[][], "Shot_OUT"=w323:T10)  [unwired: 7 in]
        }
        n122 = Bundle By Name(cluster=w316, "InitCluster.ShotArray"=w315, "InitCluster.IntensityArray"=w314) -> (w313:T18)
        n123 = call <vilib>:"Add State(s) to Queue__JKI_lib_State_Machine.vi"("State(s) in (\"\")"=w321) -> ("States Out"=w320:string)  [unwired: 14 in]
      }
      frame "SHOOT_SHIP" {
        n124 = Unbundle By Name(w343) -> ("InitCluster.ShotArray"=w340:T10[], "InitCluster.Spaceship.Shot.Speed"=w330:u32, "InitCluster.Spaceship.Shot.Length"=w327:u32, "InitCluster.Spaceship.Shot.Width"=w334:u32, "SpaceshipPosition.right"=w338:i16, "SpaceshipPosition.left"=w337:i16, "SpaceshipPosition.top"=w331:i16)
        n125 = call "FindMiddlePoint.vi"("left"=w337, "right"=w338) -> ("middle"=w335:dbl)  [unwired: 3 in]
        n126 = Subtract(x=w331, y=w330) -> (x-y=w328:u32)
        n127 = Add(x=w335, y=w334) -> (x+y=w336:dbl)
        n128 = Add(x=w327, y=w328) -> (x+y=w329:u32)
        n129 = Bundle By Name(cluster=T10 {"Speed"=0, "Length"=0, "Width"=0, "Position"={"left"=0, "top"=0, "right"=0, "bottom"=0}, "Direction"=enum."up"} ("Shot"), "Speed"=w330, "Length"=w327, "Width"=w334, "Direction"=move_dir_ud."up", "Position.left"=w335, "Position.top"=w328, "Position.right"=w336, "Position.bottom"=w329) -> (w333:T10)
        n130 = Build Array (concatenate)(w340, w333) -> (w339:T10[])
        n131 = Bundle By Name(cluster=w343, "InitCluster.ShotArray"=w339) -> (w332:T18)
        n132 = call <vilib>:"Add State(s) to Queue__JKI_lib_State_Machine.vi"("State(s) in (\"\")"=w346) -> ("States Out"=w345:string)  [unwired: 14 in]
      }
      frame "CHECK_SHOTS" {
        n133 = Unbundle By Name(w349) -> ("SpaceshipPosition"=w358:T19, "InvaderPosArray"=w361:T8, "InitCluster.ShotArray"=w353:T10[], "InitCluster.IntensityArray"=w352:u8[][])  [unwired: 1 out]
        n134 = call "CheckShot2Shot.vi"("IntensityArray_IN"=w352, "ShotArray_IN"=w353) -> ("ShotArray_OUT"=w362:T10[], "IntensityArray_OUT"=w351:u8[][])  [unwired: 8 in]
        n135 = call "CheckShot2Invader_new.vi"("IntensityArray_IN"=w351, "InvaderPosArray_IN"=w361, "ShotArray_IN"=w362) -> ("ShotArray_OUT"=w359:T10[], "IntensityArray_OUT"=w348:u8[][], "InvaderPosArray_OUT"=w360:T8)  [unwired: 6 in]
        n136 = call "CheckShots2Ship.vi"("IntensityArray_IN"=w348, "SpaceshipPosition"=w358, "ShotArray_IN"=w359) -> ("ShotArray_OUT"=w357:T10[], "IntensityArray_OUT"=w347:u8[][], "GameOver"=w355:bool)  [unwired: 6 in]
        n137 = case shown="True" w355 {
          tunnel: ["" ("State with Arguments") w368] -> w354
          frame False {
          }
          frame True {
            n138 = call <vilib>:"Build State String with Arguments__JKI_lib_State_Machine.vi"("Arguments (\"\")"="SHIP" ("Arguments (\"\")"), "State"="CHECK_END") -> ("State with Arguments"=w368:string)  [unwired: 4 in]
          }
        }
        n139 = call "CheckShot2Boundary.vi"("IntensityArray_IN"=w347, "ShotArray_IN"=w357) -> ("ShotArray_OUT"=w356:T10[], "IntensityArray_OUT"=w350:u8[][])  [unwired: 8 in]
        n140 = Bundle By Name(cluster=w349, "InvaderPosArray"=w360, "InitCluster.ShotArray"=w356, "InitCluster.IntensityArray"=w350) -> (w363:T18)
        n141 = call <vilib>:"Add State(s) to Queue__JKI_lib_State_Machine.vi"("State(s) in (\"\")"=w366, "State(s) at Back (\"\")"=w354) -> ("States Out"=w365:string)  [unwired: 13 in]
      }
      frame "CHECK_END" {
        n142 = Unbundle By Name(w376) -> ("InvaderPosArray.InvaderAlive"=w375:bool[][])
        n143 = Or Array Elements(Boolean array=w375) -> (logical OR=w374:bool)
        n144 = case shown="True" w374 {
          tunnel: [w380 w391] -> w371
          tunnel: w373 -> [w381 _]
          tunnel: w372 -> [w379 _]
          frame True {
            n145 = case shown="\"SHIP\"" w381 {
              tunnel: [w382 w383] -> w380
              tunnel: w379 -> [w382 _]
              frame Default {
              }
              frame "SHIP" {
                n146 = Two Button Dialog(message="GAME OVER\nYou couldn't save  EARTH!\nAnother invasion?", 1:"NO" ("F button name (\"Cancel\")"), 2:"YES" ("T button name (\"OK\")")) -> (T button?=w389:bool)
                n147 = Select(t="Macro: Initialize", s=w389, f="Macro: Exit") -> (s? t:f=w383:string)
              }
            }
          }
          frame False {
            n148 = Two Button Dialog(message="You saved EARTH!\nAnother invasion?", 1:"NO" ("F button name (\"Cancel\")"), 2:"YES" ("T button name (\"OK\")")) -> (T button?=w396:bool)
            n149 = Select(t="Macro: Initialize", s=w396, f="Macro: Exit") -> (s? t:f=w391:string)
          }
        }
        n150 = call <vilib>:"Add State(s) to Queue__JKI_lib_State_Machine.vi"("State(s) in (\"\")"=w371) -> ("States Out"=w378:string)  [unwired: 14 in]
      }
    }
  }
